vi "Queue Driver.vi"(0 "State":string, 5 "Data":variant, 11 "error in (no error)":errorcluster, 13 "Operation":T1=enum."Enqueue") -> (4 "State Out":string, 6 "Data Out":variant, 15 "error out":errorcluster)   [LabVIEW 2014, in "Coding Platform.lvlib"]
uses:
  Coding Platform.lvlib
  Typedefs/Queue Data.ctl
  Typedefs/Queue Driver Operations.ctl
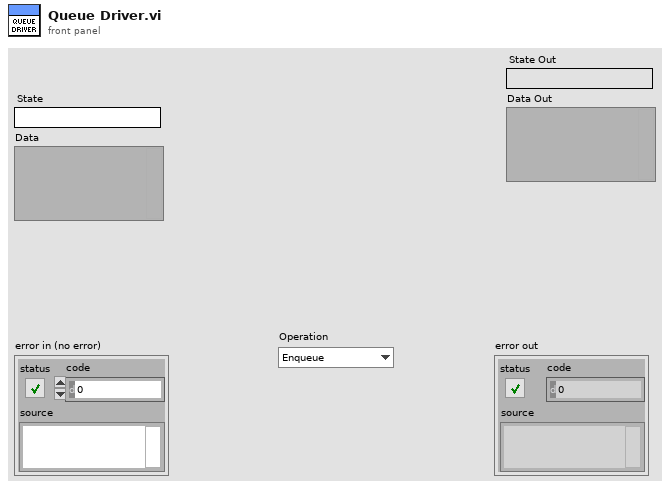
[diagram p1: front panel]
types:
  T1 = typedef "Coding Platform.lvlib/Queue Driver Operations.ctl" = enum16{"Create", "Enqueue", "Dequeue", "Destory"}
  T2 = typedef "Coding Platform.lvlib/Queue Data.ctl" = cluster{"State":string, "Data":variant}
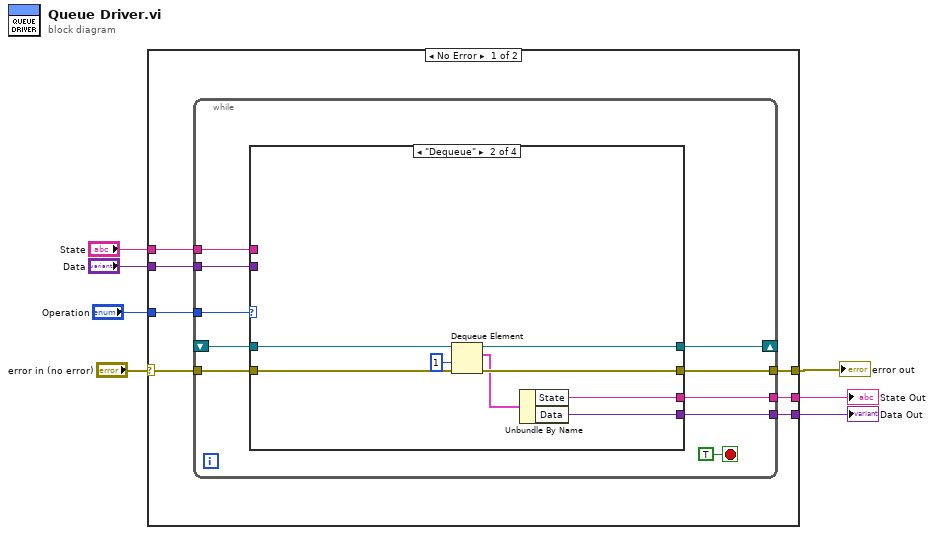
[diagram p0: block diagram]
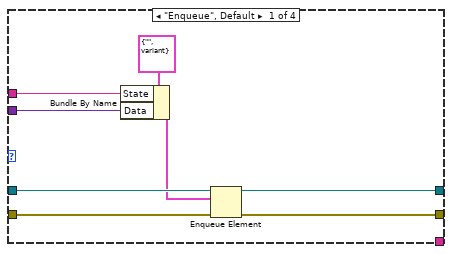
[diagram p2: hidden frame]
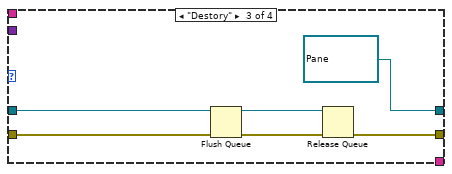
[diagram p3: hidden frame]
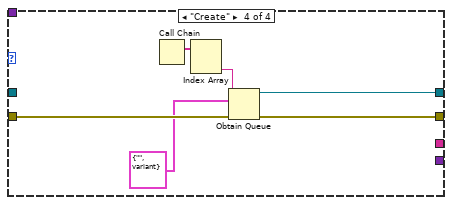
[diagram p4: hidden frame]
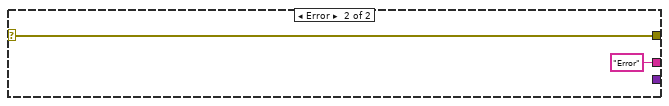
[diagram p5: hidden frame]
diagram:
  n1 = case shown="No Error" "error in (no error)" {
    selector: "error in (no error)" -> [w13 w54]
    tunnel: [w14 w54] -> w6
    tunnel: "Operation" -> [w12 _]
    tunnel: "Data" -> [w11 _]
    tunnel: "State" -> [w10 _]
    tunnel: [w9 _] -> w2
    tunnel: [w8 "Error" ("State")] -> w1
    frame No Error {
      n2 = while {
        tunnel: [w22] -> w14
        tunnel: w13 -> [w23]
        shift-right: [w21] -> _
        shift-left: _ -> [w20]
        tunnel: w12 -> [w19]
        tunnel: w11 -> [w18]
        tunnel: w10 -> [w17]
        tunnel: [w16] -> w9
        tunnel: [w15] -> w8
        stop <- TRUE ("Boolean") stop-if-true
        n3 = case shown="\"Dequeue\"" w19 {
          tunnel: w23 -> [w32 w40 w46 w52]
          tunnel: [w31 w39 w43 w51] -> w22
          tunnel: [w29 w37 refnum<queue> refnum ("queue out") w47] -> w21
          tunnel: w20 -> [w30 w38 w44 _]
          tunnel: w18 -> [w26 _ _ _]
          tunnel: w17 -> [w25 _ _ _]
          tunnel: [_ w35 _ _] -> w16
          tunnel: [_ w34 _ _] -> w15
          frame "Enqueue", Default {
            n4 = Bundle By Name(cluster=T2 {"State"="", "Data"=variant} ("element"), "State"=w25, "Data"=w26) -> (w27:T2)
            n5 = Enqueue Element(queue=w30, element=w27, error in (no error)=w32) -> (queue out=w29:refnum<queue>, error out=w31:errorcluster)  [unwired: 1 in, 1 out]
          }
          frame "Dequeue" {
            n6 = Dequeue Element(queue=w38, timeout in ms (-1)=1, error in (no error)=w40) -> (queue out=w37:refnum<queue>, element=w36:T2, error out=w39:errorcluster)  [unwired: 1 out]
            n7 = Unbundle By Name(w36) -> ("State"=w34:string, "Data"=w35:variant)
          }
          frame "Destory" {
            n8 = Flush Queue(queue=w44, error in (no error)=w46) -> (queue out=w42:refnum<queue>, error out=w45:errorcluster)  [unwired: 1 out]
            n9 = Release Queue(queue=w42, error in (no error)=w45) -> (error out=w43:errorcluster)  [unwired: 1 in, 2 out]
          }
          frame "Create" {
            n10 = Call Chain() -> (call chain=w50:string[])
            n11 = Index Array(array=w50) -> (element #2=w49:string)  [unwired: 2 in, 1 out]
            n12 = Obtain Queue(name (unnamed)=w49, element data type=T2 {"State"="", "Data"=variant}, error in (no error)=w52) -> (queue out=w47:refnum<queue>, error out=w51:errorcluster)  [unwired: 2 in, 1 out]
          }
        }
      }
    }
    frame Error {
    }
  }
  "error out" <- w6
  "State Out" <- w1
  "Data Out" <- w2
